vi "Auto Stop Tasks.vi"(8 "error in":errorcluster, 11 "All Input Tasks in":T1) -> (0 "error out":errorcluster)   [LabVIEW 2017]
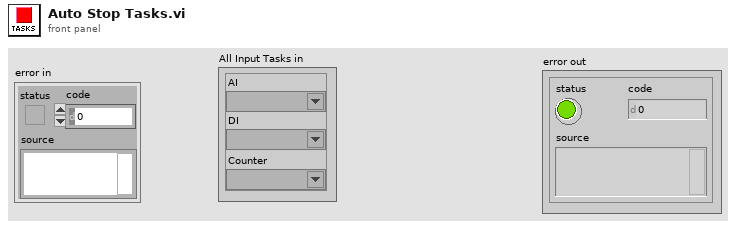
[diagram p1: front panel]
types:
  T1 = cluster{"AI":refnum<k21>, "DI":refnum<k21>, "Counter":refnum<k21>}
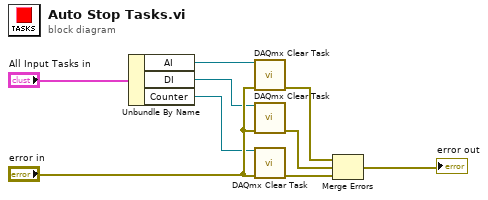
[diagram p0: block diagram]
diagram:
  n1 = Unbundle By Name("All Input Tasks in") -> ("AI"=w3:refnum<k21>, "DI"=w2:refnum<k21>, "Counter"=w1:refnum<k21>)
  n2 = call <vilib>:"DAQmx Clear Task.vi"("task in"=w3, "error in"="error in") -> ("error out"=w8:errorcluster)  [unwired: 13 in]
  n3 = call <vilib>:"DAQmx Clear Task.vi"("task in"=w2, "error in"="error in") -> ("error out"=w7:errorcluster)  [unwired: 13 in]
  n4 = call <vilib>:"DAQmx Clear Task.vi"("task in"=w1, "error in"="error in") -> ("error out"=w6:errorcluster)  [unwired: 13 in]
  n5 = Merge Errors(w8, w7, w6) -> (→"error out":errorcluster)
